vi "m1m3_logEvent_InterlockStatus.vi"(8 "error in (no error)":errorcluster, 11 "logevent_InterlockStatus_Ctl":T1) -> (0 "error out":errorcluster, 2 "function return":i32, 3 "logevent_InterlockStatus_Ctl out":T1)   [LabVIEW 2016, in "SALLV_m1m3.lvlib"]
doc: "int m1m3_shm_logEvent_InterlockStatusLV(m1m3_logevent_InterlockStatusLV *logevent_InterlockStatus_Ctl );"
uses:
  SALLV_m1m3.lvlib
  DataTypes/logevent_InterlockStatus.ctl
  SALLV_m1m3.so
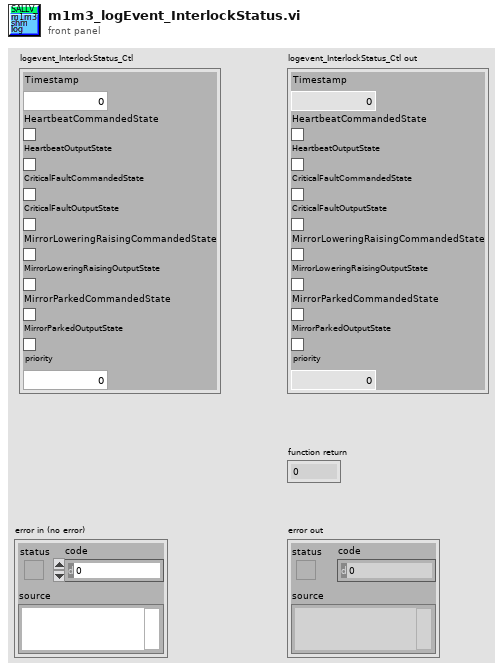
[diagram p1: front panel]
types:
  T1 = typedef "SALLV_m1m3.lvlib/logevent_InterlockStatus.ctl" = cluster{"Timestamp":dbl, "HeartbeatCommandedState":bool, "HeartbeatOutputState":bool, "CriticalFaultCommandedState":bool, "CriticalFaultOutputState":bool, "MirrorLoweringRaisingCommandedState":bool, "MirrorLoweringRaisingOutputState":bool, "MirrorParkedCommandedState":bool, "MirrorParkedOutputState":bool, "priority":i32}
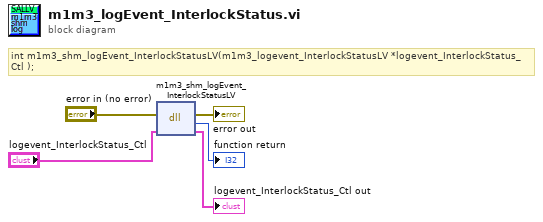
[diagram p0: block diagram]
diagram:
  # "int m1m3_shm_logEvent_InterlockStatusLV(m1m3_logevent_InterlockStatusLV *logevent_InterlockStatus_Ctl );"
  n1 = dll-call lib="opt/CODE/SALLV_m1m3/SALLV_m1m3.*" fn="m1m3_shm_logEvent_InterlockStatusLV"(error in="error in (no error)", "logevent_InterlockStatus_Ctl"="logevent_InterlockStatus_Ctl") -> (error out=→"error out":errorcluster, →"function return":i32, "logevent_InterlockStatus_Ctl"=→"logevent_InterlockStatus_Ctl out":T1)  [unwired: 2 in, 1 out]
